vi "Publish Data.vi"(8 "error in (no error)":errorcluster, 10 "waveform":waveform(dbl)[](array[waveform]), 11 "Device in":refnum<class "Device.lvclass">) -> (0 "error out":errorcluster, 3 "Device out":refnum<class "Device.lvclass">)   [LabVIEW 2023, in "Device.lvlib" / "Device.lvclass"]
uses:
  Device.lvclass
  Device.lvclass/Device.ctl
  Accessor/Get Device Name.vi
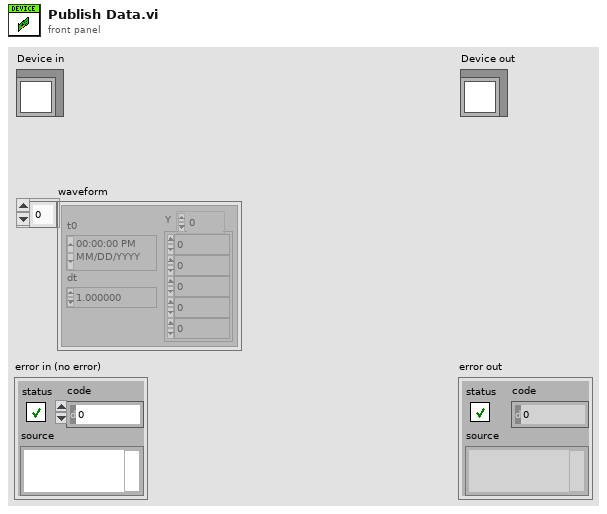
[diagram p1: front panel]
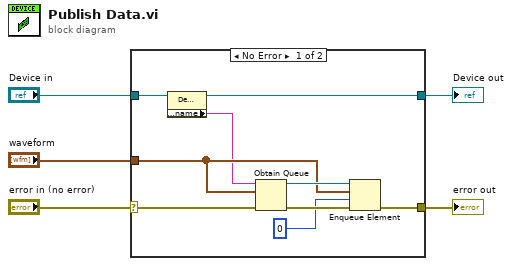
[diagram p0: block diagram]
diagram:
  n1 = case shown="No Error" "error in (no error)" {
    selector: "error in (no error)" -> [w14 w16]
    tunnel: [w9 w16] -> w4
    tunnel: [w7 w15] -> w2
    tunnel: "Device in" -> [w8 w15]
    tunnel: "waveform" -> [w10 _]
    frame No Error {
      n2 = property class="Device.lvclass"(reference=w8) -> (reference out=w7:refnum<class "Device.lvclass">, "Accessor:name"=w6:string)  [unwired: 1 in, 1 out]
      n3 = Obtain Queue(name (unnamed)=w6, element data type=w10, error in (no error)=w14) -> (queue out=w12:refnum<queue>, error out=w13:errorcluster)  [unwired: 2 in, 1 out]
      n4 = Enqueue Element(queue=w12, element=w10, timeout in ms (-1)=0, error in (no error)=w13) -> (error out=w9:errorcluster)  [unwired: 2 out]
    }
    frame Error {
    }
  }
  "error out" <- w4
  "Device out" <- w2
